vi "_dBm_to_W.vi"(1 "Power dBm":dbl[](array[numeric])) -> (0 "Power W":dbl[](array[numeric]))   [LabVIEW 2013]
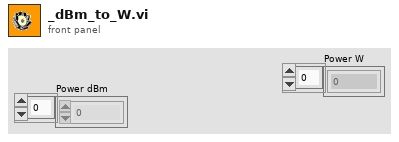
[diagram p1: front panel]
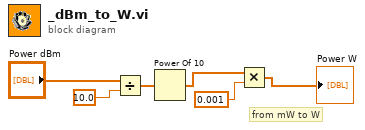
[diagram p0: block diagram]
diagram:
  # "from mW to W"
  n1 = Divide(x="Power dBm", y=10.0) -> (x/y=w6:dbl[])
  n2 = Power Of 10(x=w6) -> (10^x=w2:dbl[])
  n3 = Multiply(x=w2, y=0.001) -> (x*y=→"Power W":dbl[])
